vi "Test.vi"() -> ()   [LabVIEW 2021]
uses:
  <resource>/objmgr/daqmx.rc
panel:
  out "names out 2":string[](array[string])
  out "names out":string
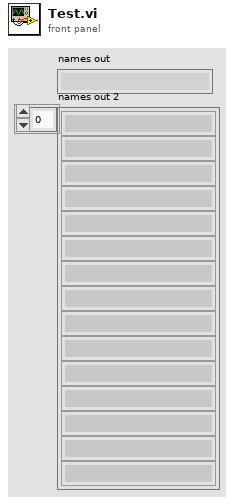
[diagram p1: front panel]
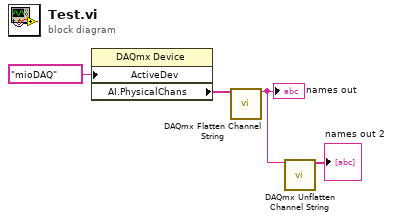
[diagram p0: block diagram]
diagram:
  n1 = property class="DAQmx Device"("ActiveDev"=tag "mioDAQ") -> ("AI.PhysicalChans"=w3:tag[])  [unwired: 2 in, 2 out]
  n2 = call <vilib>:"DAQmx Flatten Channel String.vi"("names in"=w3) -> ("names out"=w1:string)  [unwired: 13 in, 1 out]
  "names out" <- w1
  n3 = call <vilib>:"DAQmx Unflatten Channel String.vi"("names in"=w1) -> ("names out"=→"names out 2":string[])  [unwired: 13 in, 1 out]
